vi "SVT UFF58 Read Spectrum (Complex).vi"(0 "function refnum":refnum<k20>, 11 "error in (no error)":errorcluster) -> (3 "ID lines (1-3)":T2, 4 "dup function refnum":refnum<k20>, 6 "real part":T1(graph), 8 "imaginary part":T1(graph), 15 "error out":errorcluster)   [LabVIEW 2017, in "SoundVib_UFF58.lvlib"]
doc: "Reads data from a UFF58 (universal file format) function specified by the <B>function refnum</B> input. This VI also reads the fields in records 1, 2, and 3, returned by ID lines (1-3). You can read a single time domain waveform, a single frequency spectrum, the real and imaginary parts of a frequency spectrum, and any data from a function. The default instance, SVT UFF58 Read Time Waveform, reads a single time domain waveform from a function specified by the <B>function refnum</B> input. Wire data to the <B>function refnum</B> input to determine the polymorphic instance to use or manually select the instance."
uses:
  <vilib>/addons/Sound and Vibration/svt_UFF58/SoundVib_UFF58.lvlib
  <vilib>/addons/Sound and Vibration/svt_UFF58/subVIs/sv_IDLines123.ctl
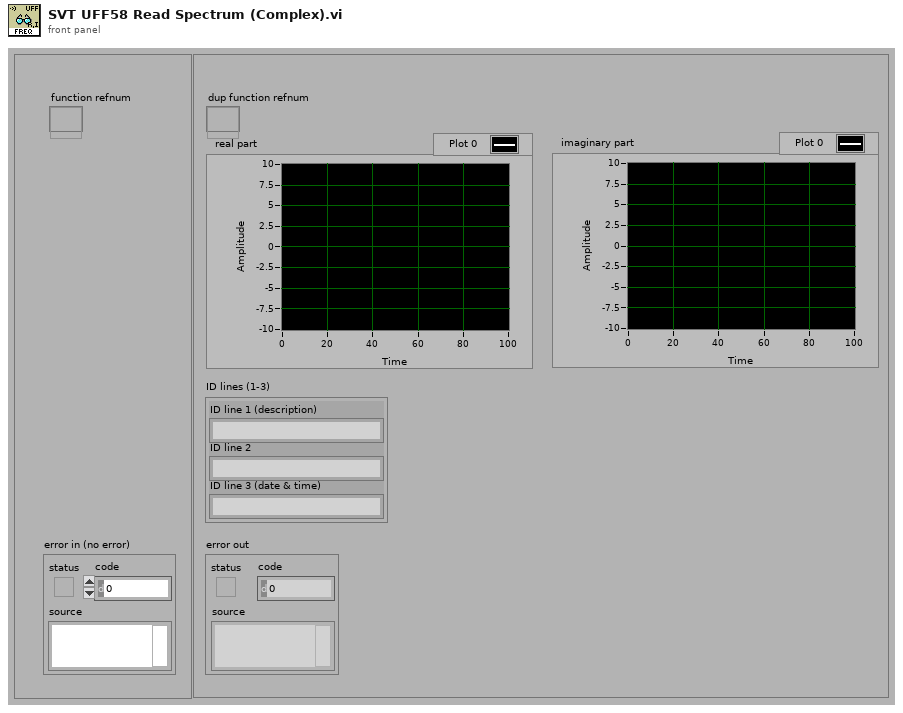
[diagram p1: front panel]
types:
  T1 = cluster{"abscissa minimum":dbl, "abscissa increment":dbl, "data":dbl[]}
  T2 = typedef "SoundVib_UFF58.lvlib/sv_IDLines123.ctl" = cluster{"ID line 1 (description)":string, "ID line 2":string, "ID line 3 (date & time)":string}
  T3 = typedef "SoundVib_UFF58.lvlib/sv_UFF58 DOF.ctl" = cluster{"function type":T4, "function ID number":i32, "version number":i32, "load case ID number":i32, "response entity name":string, "response node":i32, "response direction":T5, "reference entity name":string, "reference node":i32, "reference direction":T5}
  T4 = typedef "SoundVib_UFF58.lvlib/sv_FunctionType.ctl" = enum16{"general or unknown", "time response", "auto spectrum", "cross spectrum", "frequency response function", "transmissibility", "coherence", "auto correlation", "cross correlation", "power spectral density (PSD)", "energy spectral density (ESD)", "probability density function", "spectrum", "cumulative frequency distribution", "peaks valley", "stress/cycles", "strain/cycles", "orbit", "mode indicator function", "force pattern", "partial power", "partial coherence", "eigenvalue", "eigenvector", "shock response spectrum", "finite impulse response filter", "multiple coherence", "order function", "phase compensation"}
  T5 = typedef "SoundVib_UFF58.lvlib/sv_UFF58 Response Direction.ctl" = i32
  T6 = typedef "SoundVib_UFF58.lvlib/sv_UFF58 Data Form.ctl" = cluster{"ordinate data type":u16, "number of data values/pairs":i32, "abscissa spacing":enum16{"uneven", "even"}, "abscissa minimum":dbl, "abscissa increment":dbl}
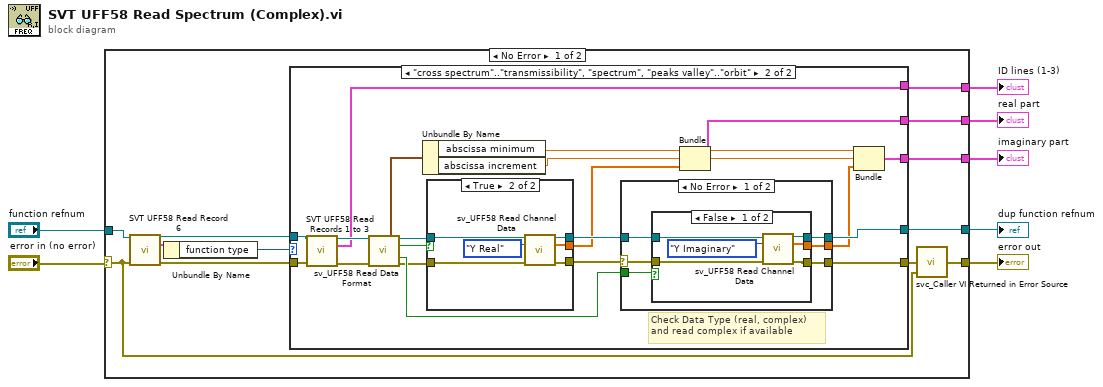
[diagram p0: block diagram]
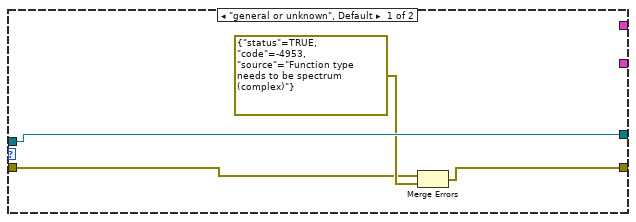
[diagram p2: hidden frame]
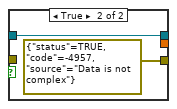
[diagram p3: hidden frame]
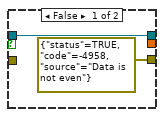
[diagram p5: hidden frame]
diagram:
  n1 = case shown="No Error" "error in (no error)" {
    selector: "error in (no error)" -> [w10 w68]
    tunnel: "function refnum" -> [w11 w69]
    tunnel: [w19 _] -> w7
    tunnel: [w14 _] -> w6
    tunnel: [w18 w69] -> w1
    tunnel: [w15 w68] -> w5
    tunnel: [w17 _] -> w4
    frame No Error {
      n2 = call <vilib>:"SVT UFF58 Read Record 6.vi"("function refnum"=w11, "error in (no error)"=w10) -> ("dup function refnum"=w9:refnum<k20>, "DOF identification"=w13:T3, "error out"=w8:errorcluster)  [unwired: 11 in]
      n3 = Unbundle By Name(w13) -> ("function type"=w12:T4)
      n4 = case shown="\"cross spectrum\"..\"transmissibility\", \"spectrum\", \"peaks valley\"..\"orbit\"" w12 {
        tunnel: [_ w41] -> w19
        tunnel: [w23 w39] -> w18
        tunnel: [_ w38] -> w17
        tunnel: [w20 w36] -> w16
        tunnel: [_ w31] -> w14
        tunnel: w9 -> [w23 w25]
        tunnel: w8 -> [w21 w24]
        frame "general or unknown", Default {
          n5 = Merge Errors(w21, errorcluster {"status"=TRUE, "code"=-4953, "source"="Function type needs to be spectrum (complex)"} ("error out")) -> (w20:errorcluster)
        }
        frame "cross spectrum".."transmissibility", "spectrum", "peaks valley".."orbit" {
          # "Check Data Type (real, complex) \nand read complex if available"
          n6 = call <vilib>:"SVT UFF58 Read Records 1 to 3.vi"("function refnum"=w25, "error in (no error)"=w24) -> ("dup function refnum"=w43:refnum<k20>, "ID lines (1-3)"=w41:T2, "error out"=w42:errorcluster)  [unwired: 11 in]
          n7 = call <vilib>:"sv_UFF58 Read Data Format.vi"("function refnum"=w43, "error in (no error)"=w42) -> ("data form"=w30:T6, "dup function refnum"=w34:refnum<k20>, "even"=w33:bool, "real"=w40:bool, "error out"=w35:errorcluster)  [unwired: 9 in]
          n8 = Unbundle By Name(w30) -> ("abscissa minimum"=w28:dbl, "abscissa increment"=w27:dbl)
          n9 = case shown="True" w33 {
            tunnel: w34 -> [w61 w64]
            tunnel: w35 -> [_ w63]
            tunnel: [w61 w66] -> w32
            tunnel: [errorcluster {"status"=TRUE, "code"=-4958, "source"="Data is not even"} ("error out") w65] -> w26
            tunnel: [_ w62] -> w29
            frame False {
            }
            frame True {
              n10 = call <vilib>:"sv_UFF58 Read Channel Data.vi"("function refnum"=w64, "channel to read"=enum16{"X", "Y Real", "Y Imaginary"}."Y Real" ("data to read"), "error in (no error)"=w63) -> ("dup function refnum"=w66:refnum<k20>, "data"=w62:dbl[], "error out"=w65:errorcluster)  [unwired: 10 in]
            }
          }
          n11 = case shown="No Error" w26 {
            selector: w26 -> [w44 w58]
            tunnel: w40 -> [w49 _]
            tunnel: [w48 w59] -> w39
            tunnel: [w47 _] -> w37
            tunnel: [w46 w58] -> w36
            tunnel: w32 -> [w45 w59]
            frame No Error {
              n12 = case shown="False" w49 {
                tunnel: w44 -> [w55 _]
                tunnel: w45 -> [w54 w57]
                tunnel: [w52 _] -> w47
                tunnel: [w51 w57] -> w48
                tunnel: [w50 errorcluster {"status"=TRUE, "code"=-4957, "source"="Data is not complex"} ("error out")] -> w46
                frame False {
                  n13 = call <vilib>:"sv_UFF58 Read Channel Data.vi"("function refnum"=w54, "channel to read"=enum16{"X", "Y Real", "Y Imaginary"}."Y Imaginary" ("data to read"), "error in (no error)"=w55) -> ("dup function refnum"=w51:refnum<k20>, "data"=w52:dbl[], "error out"=w50:errorcluster)  [unwired: 10 in]
                }
                frame True {
                }
              }
            }
            frame Error {
            }
          }
          n14 = Bundle("abscissa minimum"=w28, "abscissa increment"=w27, "data"=w29) -> (w31:T1)  [unwired: 1 in]
          n15 = Bundle("abscissa minimum"=w28, "abscissa increment"=w27, "data"=w37) -> (w38:T1)  [unwired: 1 in]
        }
      }
      n16 = call <vilib>:"svc_Caller VI Returned in Error Source.vi"("warning input to caller"=w10, "error in (no error)"=w16) -> ("error out"=w15:errorcluster)  [unwired: 3 in]
    }
    frame Error {
    }
  }
  "error out" <- w5
  "ID lines (1-3)" <- w7
  "real part" <- w6
  "imaginary part" <- w4
  "dup function refnum" <- w1
